vi "RP-VNA DATA TBL Extract.vi"(4 "VNA DATA CLUSTER TBL":T1(array[cluster]), 5 "index":i32) -> (1 "appended array":ext[][](array[numeric]), 2 "CHANNEL":dbl)   [LabVIEW 2021]
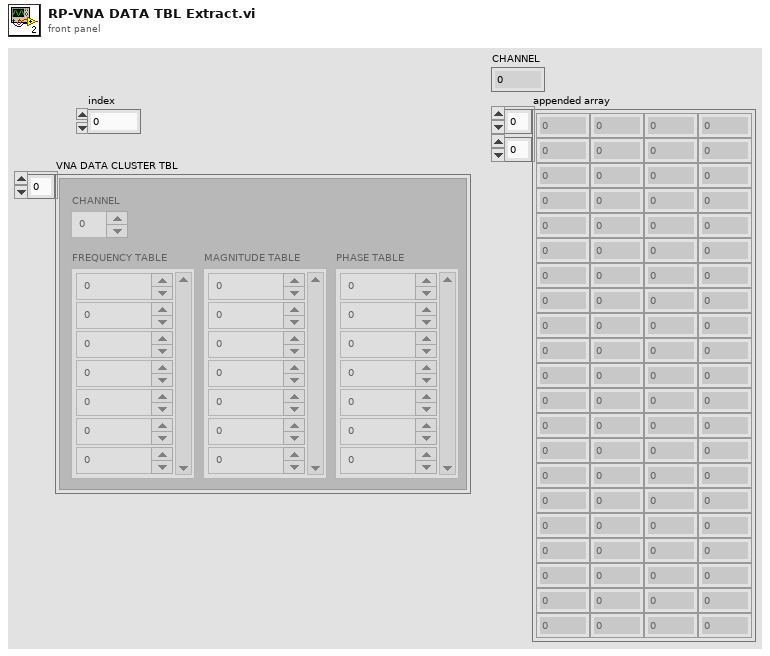
[diagram p1: front panel]
types:
  T1 = cluster{"CHANNEL":dbl, "FREQUENCY TABLE":ext[], "MAGNITUDE TABLE":ext[], "PHASE TABLE":ext[]}[]
  T2 = cluster{"CHANNEL":dbl, "FREQUENCY TABLE":ext[], "MAGNITUDE TABLE":ext[], "PHASE TABLE":ext[]}
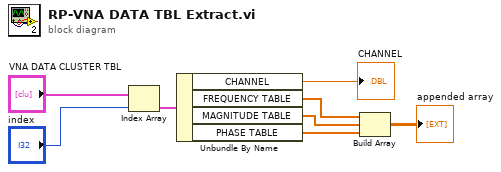
[diagram p0: block diagram]
diagram:
  n1 = Index Array(array="VNA DATA CLUSTER TBL", index="index") -> (element=w6:T2)
  n2 = Unbundle By Name(w6) -> ("CHANNEL"=→"CHANNEL":dbl, "FREQUENCY TABLE"=w5:ext[], "MAGNITUDE TABLE"=w4:ext[], "PHASE TABLE"=w3:ext[])
  n3 = Build Array(w5, w4, w3) -> (→"appended array":ext[][])
